vi "Poll Prompt.vi"(8 "error in (no error)":errorcluster) -> (0 "error out":errorcluster, 2 "Period":i32)   [LabVIEW 2020, in "Monitored Actor.lvlib" / "Classic Monitor.lvclass"]
uses:
  <vilib>/MGI/Monitored Actor/Classic Monitor/Monitor/Monitor Actor/Classic Monitor.lvclass
panel:
  in  "OK":bool
  in  "Poll Period":i32=1000 caption="ms"
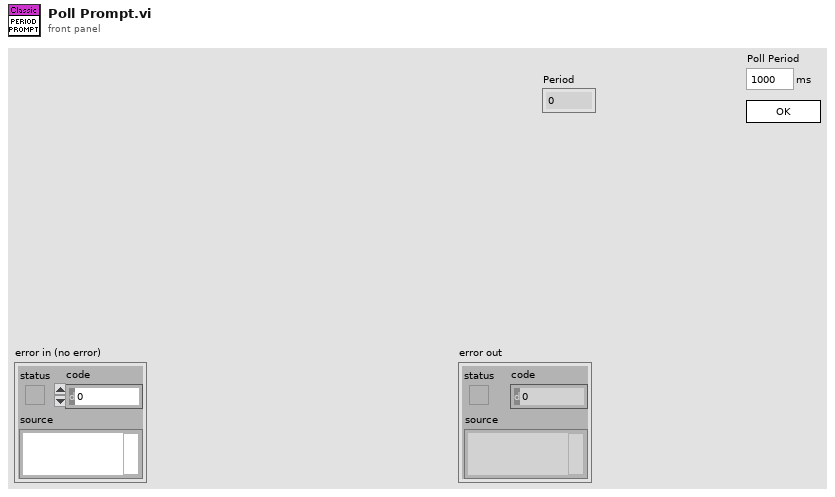
[diagram p1: front panel]
types:
  T1 = enum32{"Invalid", "Standard", "Closed", "Hidden", "Minimized", "Maximized"}
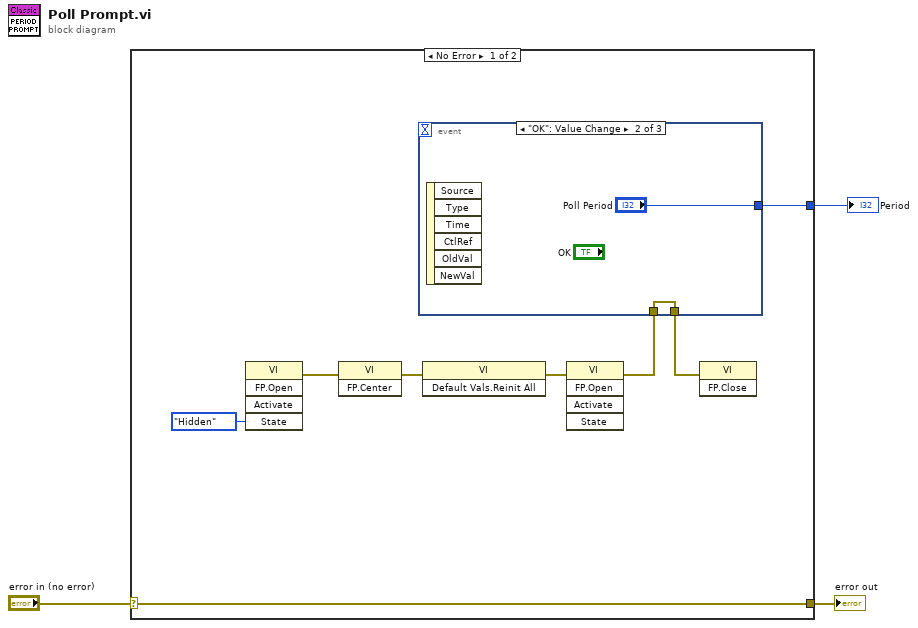
[diagram p0: block diagram]
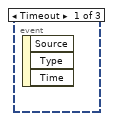
[diagram p2: hidden frame]
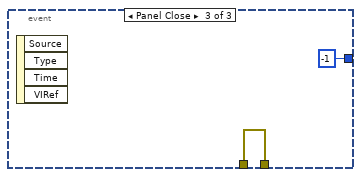
[diagram p3: hidden frame]
diagram:
  n1 = case shown="No Error" "error in (no error)" {
    selector: "error in (no error)" -> [w11 w16]
    tunnel: [w11 w16] -> w2
    tunnel: [w10 _] -> w1
    frame No Error {
      n2 = invoke class="VI" method="FP.Open"("State"=T1."Hidden") -> (error out=w8:errorcluster)  [unwired: 4 in, 4 out]
      n3 = invoke class="VI" method="FP.Center"(error in=w8) -> (error out=w7:errorcluster)  [unwired: 2 in, 2 out]
      n4 = invoke class="VI" method="Default Vals.Reinit All"(error in=w7) -> (error out=w6:errorcluster)  [unwired: 2 in, 2 out]
      n5 = invoke class="VI" method="FP.Open"(error in=w6) -> (error out=w5:errorcluster)  [unwired: 4 in, 4 out]
      n6 = event shown="[1] \"OK\": Value Change" {
        selector: _ -> [_ _ _]
        dyn-events: _ -> [_ _ _]
        timeout: _ -> [_ _ _]
        tunnel: [_ "Poll Period" -1 ("Poll Period")] -> w10
        tunnel: [_ w12 w14] -> w4
        tunnel: w5 -> [_ w12 w14]
        event Timeout {
          n7 = event-data() -> ()  [unwired: 1 in, 3 out]
        }
        event "OK": Value Change {
          n8 = event-data() -> ()  [unwired: 1 in, 6 out]
        }
        event Panel Close {
          n9 = event-data() -> ()  [unwired: 1 in, 4 out]
        }
      }
      n10 = invoke class="VI" method="FP.Close"(error in=w4) -> ()  [unwired: 2 in, 3 out]
    }
    frame Error {
    }
  }
  "error out" <- w2
  "Period" <- w1
